vi "SCS IPG Charging Station.vi"() -> ()   [LabVIEW 2020]
uses:
  Charger_Status Control.ctl
  Drivers/Charger Test Set/Charger_Input Control.ctl
  MICS_Input Control.ctl
  Drivers/Charging/Charging_MICS Retry Count.vi
panel:
  in  "RUN":bool
  in  "PRINT":bool
  in  "VBAT":bool
  out "IPG 6":T1={"MICS ID"=0, "VBAT"=nan, "ChargingState"="", "VBAT Slide"=3.5, "Status"="Ready to Load Fixture.", "TemperatureLevel"=nan, "IPG_ReceivedLevel"=nan, "VBAT Target"=0.0, "Charger Setpoint"=7500.0, "Index"=0, "Ready"=TRUE, "Charger Inputs"={"address"="COM17", "position"=0, "setpoint"=7500.0}, "MICS Inputs"={"address"="COM17", "chan"=0, "ID"=0}} {"MICS Inputs"."ID" format="%06x"; "MICS Inputs"."chan" min=1 max=10 step=1; "Charger Inputs"."setpoint" min=0.0 max=20000.0 step=100.0; "Charger Inputs"."position" min=0 max=5 step=1; "MICS ID" format="%06x"; "VBAT Target" format="%.2f"; "VBAT Slide" scale=3.5..4.0 scale format="%.2f"; "VBAT" format="%.2f"}
  out "IPG 5":T1={"MICS ID"=0, "VBAT"=nan, "ChargingState"="", "VBAT Slide"=3.5, "Status"="Ready to Load Fixture.", "TemperatureLevel"=nan, "IPG_ReceivedLevel"=nan, "VBAT Target"=0.0, "Charger Setpoint"=7500.0, "Index"=0, "Ready"=TRUE, "Charger Inputs"={"address"="COM17", "position"=0, "setpoint"=7500.0}, "MICS Inputs"={"address"="COM17", "chan"=0, "ID"=0}} {"MICS Inputs"."ID" format="%06x"; "MICS Inputs"."chan" min=1 max=10 step=1; "Charger Inputs"."setpoint" min=0.0 max=20000.0 step=100.0; "Charger Inputs"."position" min=0 max=5 step=1; "MICS ID" format="%06x"; "VBAT Target" format="%.2f"; "VBAT Slide" scale=3.5..4.0 scale format="%.2f"; "VBAT" format="%.2f"}
  in  "STOP":bool
  out "IPG 4":T1={"MICS ID"=0, "VBAT"=nan, "ChargingState"="", "VBAT Slide"=3.5, "Status"="Ready to Load Fixture.", "TemperatureLevel"=nan, "IPG_ReceivedLevel"=nan, "VBAT Target"=0.0, "Charger Setpoint"=7500.0, "Index"=0, "Ready"=TRUE, "Charger Inputs"={"address"="COM17", "position"=0, "setpoint"=7500.0}, "MICS Inputs"={"address"="COM17", "chan"=0, "ID"=0}} {"MICS Inputs"."ID" format="%06x"; "MICS Inputs"."chan" min=1 max=10 step=1; "Charger Inputs"."setpoint" min=0.0 max=20000.0 step=100.0; "Charger Inputs"."position" min=0 max=5 step=1; "MICS ID" format="%06x"; "VBAT Target" format="%.2f"; "VBAT Slide" scale=3.5..4.0 scale format="%.2f"; "VBAT" format="%.2f"}
  out "IPG 3":T1={"MICS ID"=0, "VBAT"=nan, "ChargingState"="", "VBAT Slide"=3.5, "Status"="Ready to Load Fixture.", "TemperatureLevel"=nan, "IPG_ReceivedLevel"=nan, "VBAT Target"=0.0, "Charger Setpoint"=7500.0, "Index"=0, "Ready"=TRUE, "Charger Inputs"={"address"="COM17", "position"=0, "setpoint"=7500.0}, "MICS Inputs"={"address"="COM17", "chan"=0, "ID"=0}} {"MICS Inputs"."ID" format="%06x"; "MICS Inputs"."chan" min=1 max=10 step=1; "Charger Inputs"."setpoint" min=0.0 max=20000.0 step=100.0; "Charger Inputs"."position" min=0 max=5 step=1; "MICS ID" format="%06x"; "VBAT Target" format="%.2f"; "VBAT Slide" scale=3.5..4.0 scale format="%.2f"; "VBAT" format="%.2f"}
  out "IPG 2":T1={"MICS ID"=0, "VBAT"=nan, "ChargingState"="", "VBAT Slide"=3.5, "Status"="Ready to Load Fixture.", "TemperatureLevel"=nan, "IPG_ReceivedLevel"=nan, "VBAT Target"=0.0, "Charger Setpoint"=7500.0, "Index"=0, "Ready"=TRUE, "Charger Inputs"={"address"="COM17", "position"=0, "setpoint"=7500.0}, "MICS Inputs"={"address"="COM17", "chan"=0, "ID"=0}} {"MICS Inputs"."ID" format="%06x"; "MICS Inputs"."chan" min=1 max=10 step=1; "Charger Inputs"."setpoint" min=0.0 max=20000.0 step=100.0; "Charger Inputs"."position" min=0 max=5 step=1; "MICS ID" format="%06x"; "VBAT Target" format="%.2f"; "VBAT Slide" scale=3.5..4.0 scale format="%.2f"; "VBAT" format="%.2f"}
  out "IPG 1":T1={"MICS ID"=0, "VBAT"=nan, "ChargingState"="", "VBAT Slide"=3.5, "Status"="Ready to Load Fixture.", "TemperatureLevel"=nan, "IPG_ReceivedLevel"=nan, "VBAT Target"=0.0, "Charger Setpoint"=7500.0, "Index"=0, "Ready"=TRUE, "Charger Inputs"={"address"="COM8", "position"=0, "setpoint"=7500.0}, "MICS Inputs"={"address"="COM9", "chan"=0, "ID"=222740}} {"MICS Inputs"."ID" format="%06x"; "MICS Inputs"."chan" min=1 max=10 step=1; "Charger Inputs"."setpoint" min=0.0 max=20000.0 step=100.0; "Charger Inputs"."position" min=0 max=5 step=1; "MICS ID" format="%06x"; "VBAT Target" format="%.2f"; "VBAT Slide" scale=3.5..4.0 scale format="%.2f"; "VBAT" format="%.2f"}
  # "50% (VBAT 3.85)"
  # "Full Charge"
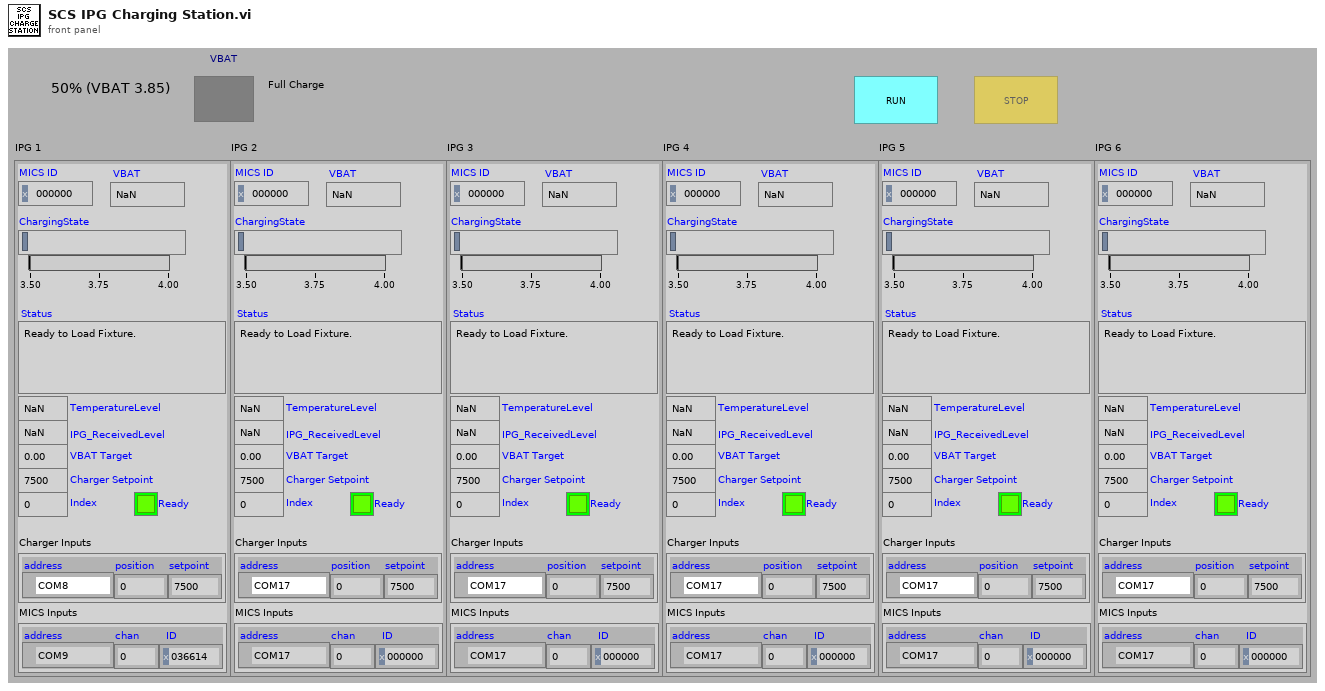
[diagram p1: front panel]
types:
  T1 = typedef "Charger_Status Control.ctl" = cluster{"MICS ID":u32, "VBAT":dbl, "ChargingState":string, "VBAT Slide":dbl, "Status":string, "TemperatureLevel":dbl, "IPG_ReceivedLevel":dbl, "VBAT Target":dbl, "Charger Setpoint":dbl, "Index":i32, "Ready":bool, "Charger Inputs":T2, "MICS Inputs":T3}
  T2 = typedef "Charger_Input Control.ctl" = cluster{"address":refnum<visa-resource-name>, "position":i32, "setpoint":dbl}
  T3 = typedef "MICS_Input Control.ctl" = cluster{"address":refnum<visa-resource-name>, "chan":u16, "ID":u32}
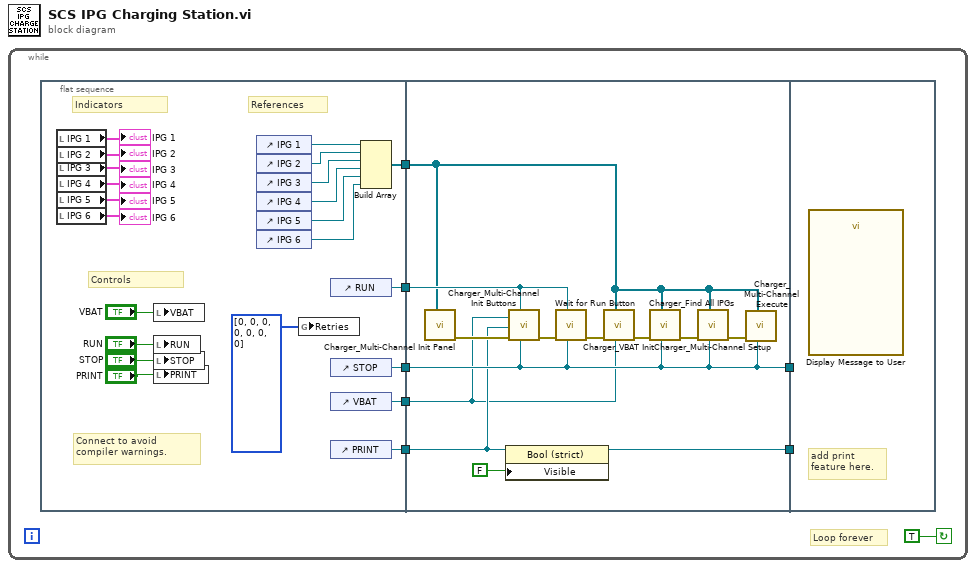
[diagram p0: block diagram]
diagram:
  n1 = while {
    stop <- TRUE continue-if-true
    # "Loop forever"
    n2 = flat-sequence {
      tunnel: [w14] -> w7
      tunnel: [w12] -> w6
      tunnel: [w13] -> w5
      tunnel: [w11] -> w8
      tunnel: [w10] -> w1
      tunnel: [w35] -> w4
      tunnel: [w39] -> w3
      tunnel: w8 -> [w36]
      tunnel: w7 -> [w31]
      tunnel: w6 -> [w39]
      tunnel: w5 -> [w42]
      tunnel: w1 -> [w32]
      tunnel: w4 -> [_]
      tunnel: w3 -> [_]
      frame #0 {
        # "References"
        # "Indicators"
        # "Controls"
        # "Connect to avoid compiler warnings."
        n3 = local read "IPG 1"() -> (→"IPG 1":T1)
        n4 = local read "IPG 2"() -> (→"IPG 2":T1)
        n5 = local read "IPG 3"() -> (→"IPG 3":T1)
        n6 = local read "IPG 4"() -> (→"IPG 4":T1)
        n7 = local read "IPG 5"() -> (→"IPG 5":T1)
        n8 = local read "IPG 6"() -> (→"IPG 6":T1)
        n9 = local write "VBAT"("VBAT") -> ()
        n10 = local write "RUN"("RUN") -> ()
        n11 = local write "STOP"("STOP") -> ()
        n12 = local write "PRINT"("PRINT") -> ()
        n13 = control-ref of="IPG 1"() -> (w15:refnum<vi>)
        n14 = control-ref of="IPG 2"() -> (w16:refnum<vi>)
        n15 = control-ref of="IPG 3"() -> (w20:refnum<vi>)
        n16 = control-ref of="IPG 4"() -> (w17:refnum<vi>)
        n17 = control-ref of="IPG 5"() -> (w18:refnum<vi>)
        n18 = control-ref of="IPG 6"() -> (w19:refnum<vi>)
        n19 = global write "Charging_MICS Retry Count.vi" "Retries"(u8[] [0, 0, 0, 0, 0, 0, 0] ("Retries")) -> ()
        n20 = control-ref of="RUN"() -> (w13:refnum<vi>)
        n21 = control-ref of="STOP"() -> (w12:refnum<vi>)
        n22 = control-ref of="VBAT"() -> (w10:refnum<vi>)
        n23 = control-ref of="PRINT"() -> (w11:refnum<vi>)
        n24 = Build Array(w15, w16, w20, w17, w18, w19) -> (w14:refnum<vi>[])
      }
      frame #1 {
        n25 = call "Charger_Multi-Channel Init Panel.vi"("Status Refnum  Array"=w31) -> ("error out"=w38:errorcluster)  [unwired: 8 in]
        n26 = property class="Bool (strict)"(reference=w36, "Visible"=FALSE) -> (reference out=w35:refnum<vi>)  [unwired: 1 in, 1 out]
        n27 = call "Charger_Multi-Channel Init Buttons.vi"("STOP refnum"=w39, "RUN refnum"=w42, "error in"=w38, "PRINT refnum"=w36, "VBAT refnum"=w32) -> ("error out"=w41:errorcluster)  [unwired: 6 in]
        n28 = call "Wait for Run Button.vi"("STOP refnum"=w39, "RUN refnum"=w42, "error in"=w41) -> ("error out"=w34:errorcluster)  [unwired: 7 in, 1 out]
        n29 = call "Charger_VBAT Init.vi"("VBAT refnum"=w32, "Status Refnum  Array"=w31, "error in"=w34) -> ("error out"=w33:errorcluster)  [unwired: 8 in]
        n30 = call "Charger_Find All IPGs.vi"("Stop Refnum"=w39, "IPG Status Array"=w31, "error in"=w33) -> ("error out"=w40:errorcluster)  [unwired: 8 in]
        n31 = call "Charger_Multi-Channel Setup.vi"("STOP Refnum"=w39, "Status Refnum  Array"=w31, "error in"=w40) -> ("error out"=w43:errorcluster)  [unwired: 8 in]
        n32 = call "Charger_Multi-Channel Execute.vi"("STOP Refnum"=w39, "Status Refnum  Array"=w31, "error in"=w43) -> ()  [unwired: 8 in, 1 out]
      }
      frame #2 {
        # "add print\nfeature here."
        n33 = call "Display Message to User"() -> ()  [unwired: 10 in, 2 out]
      }
    }
  }
